vi "Asylum_ReadScanSizeAndOffset.vi"(11 "Read in the string file":string) -> (0 "Y Offset":dbl, 1 "X Offset":dbl, 2 "Y Range":dbl, 3 "X Range":dbl)   [LabVIEW 2020]
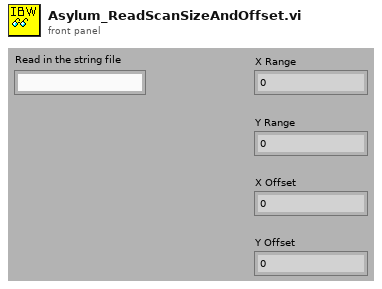
[diagram p1: front panel]
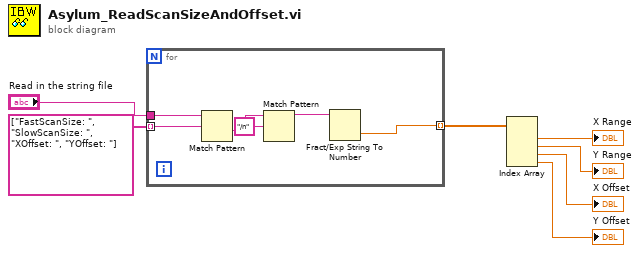
[diagram p0: block diagram]
diagram:
  n1 = for {
    tunnel: string[] ["FastScanSize: ", "SlowScanSize: ", "XOffset: ", "YOffset: "] -> [w13] mode=indexing
    tunnel: "Read in the string file" -> [w12]
    tunnel: [w9] -> w6 mode=indexing
    n2 = Match Pattern(string=w12, regular expression=w13) -> (after substring=w11:string)  [unwired: 1 in, 3 out]
    n3 = Match Pattern(string=w11, regular expression="/n") -> (before substring=w10:string)  [unwired: 1 in, 3 out]
    n4 = Fract/Exp String To Number(string=w10) -> (number=w9:dbl)  [unwired: 3 in, 1 out]
  }
  n5 = Index Array(array=w6) -> (element #1=→"X Range":dbl, element #2=→"Y Range":dbl, element #3=→"X Offset":dbl, element #4=→"Y Offset":dbl)  [unwired: 4 in]
